vi "请求参数.vi"(10 "业务参数":T1, 11 "系统参数":T2) -> (3 "已排序的数组":T3[](array[typedef]))   [LabVIEW 2016, in "Alarm interface.lvlib" / "短信语音库.lvlib"]
uses:
  <vilib>/LVH/i3 OAuth/Controls/Name-Value Pair.ctl
  <vilib>/LVH/i3 OAuth/i3-oauth.lvlib
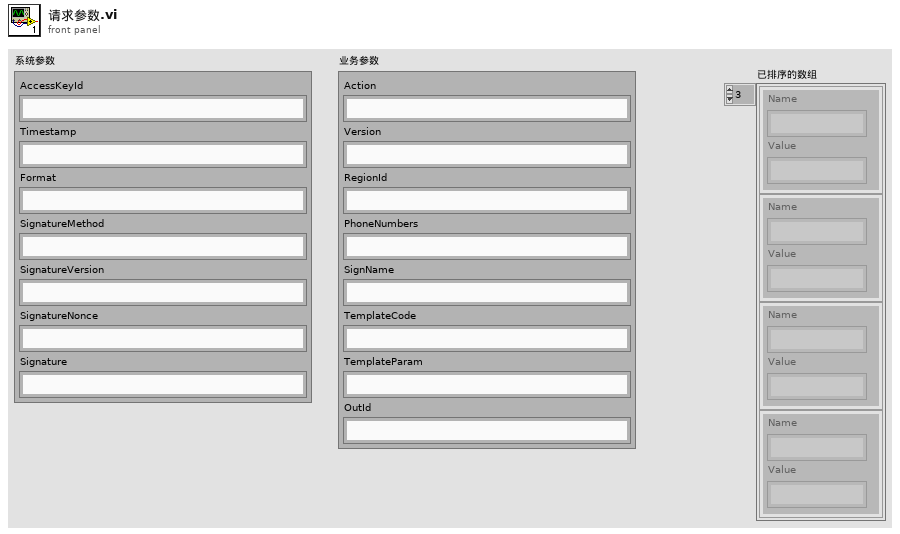
[diagram p1: front panel]
types:
  T1 = cluster{"Action":string, "Version":string, "RegionId":string, "PhoneNumbers":string, "SignName":string, "TemplateCode":string, "TemplateParam":string, "OutId":string}
  T2 = cluster{"AccessKeyId":string, "Timestamp":string, "Format":string, "SignatureMethod":string, "SignatureVersion":string, "SignatureNonce":string, "Signature":string}
  T3 = typedef "i3-oauth.lvlib/Name-Value Pair.ctl" = cluster{"Name":string, "Value":string}
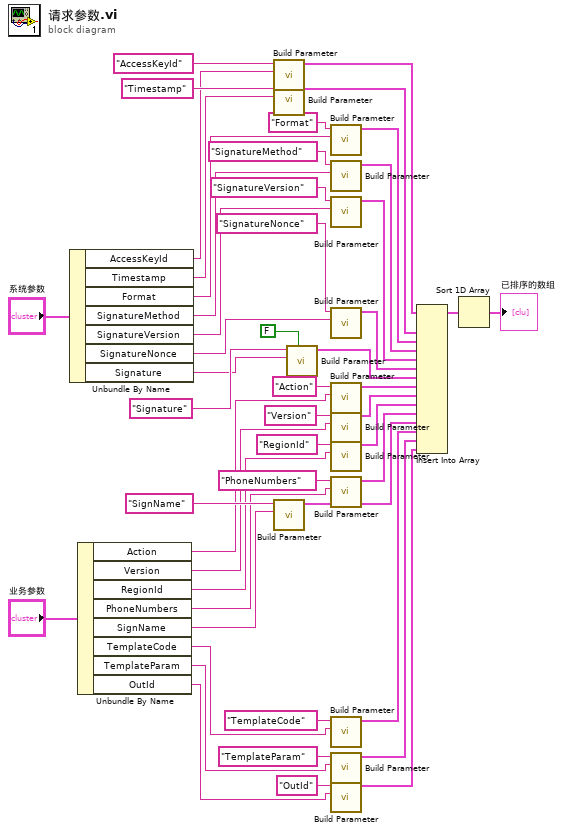
[diagram p0: block diagram]
diagram:
  n1 = Unbundle By Name("系统参数") -> ("AccessKeyId"=w25:string, "Timestamp"=w24:string, "Format"=w23:string, "SignatureMethod"=w22:string, "SignatureVersion"=w21:string, "SignatureNonce"=w20:string, "Signature"=w19:string)
  n2 = Unbundle By Name("业务参数") -> ("Action"=w14:string, "Version"=w13:string, "RegionId"=w12:string, "PhoneNumbers"=w11:string, "SignName"=w10:string, "TemplateCode"=w9:string, "TemplateParam"=w8:string, "OutId"=w7:string)
  n3 = call <vilib>:"Build Parameter.vi"("Value"=w25, "Key"="AccessKeyId") -> ("Parameter Array"=w35:T3[])  [unwired: 9 in]
  n4 = call <vilib>:"Build Parameter.vi"("Value"=w24, "Key"="Timestamp") -> ("Parameter Array"=w34:T3[])  [unwired: 9 in]
  n5 = call <vilib>:"Build Parameter.vi"("Value"=w10, "Key"="SignName") -> ("Parameter Array"=w4:T3[])  [unwired: 9 in]
  n6 = call <vilib>:"Build Parameter.vi"("Return Parameter? (T)"=FALSE, "Value"=w19, "Key"="Signature") -> ("Parameter Array"=w29:T3[])  [unwired: 8 in]
  n7 = call <vilib>:"Build Parameter.vi"("Value"=w23, "Key"="Format") -> ("Parameter Array"=w33:T3[])  [unwired: 9 in]
  n8 = call <vilib>:"Build Parameter.vi"("Value"=w22, "Key"="SignatureMethod") -> ("Parameter Array"=w32:T3[])  [unwired: 9 in]
  n9 = call <vilib>:"Build Parameter.vi"("Value"=w21, "Key"="SignatureVersion") -> ("Parameter Array"=w31:T3[])  [unwired: 9 in]
  n10 = call <vilib>:"Build Parameter.vi"("Value"=w20, "Key"="SignatureNonce") -> ("Parameter Array"=w30:T3[])  [unwired: 9 in]
  n11 = call <vilib>:"Build Parameter.vi"("Value"=w14, "Key"="Action") -> ("Parameter Array"=w18:T3[])  [unwired: 9 in]
  n12 = call <vilib>:"Build Parameter.vi"("Value"=w13, "Key"="Version") -> ("Parameter Array"=w17:T3[])  [unwired: 9 in]
  n13 = call <vilib>:"Build Parameter.vi"("Value"=w12, "Key"="RegionId") -> ("Parameter Array"=w16:T3[])  [unwired: 9 in]
  n14 = call <vilib>:"Build Parameter.vi"("Value"=w11, "Key"="PhoneNumbers") -> ("Parameter Array"=w5:T3[])  [unwired: 9 in]
  n15 = call <vilib>:"Build Parameter.vi"("Value"=w9, "Key"="TemplateCode") -> ("Parameter Array"=w3:T3[])  [unwired: 9 in]
  n16 = call <vilib>:"Build Parameter.vi"("Value"=w8, "Key"="TemplateParam") -> ("Parameter Array"=w2:T3[])  [unwired: 9 in]
  n17 = call <vilib>:"Build Parameter.vi"("Value"=w7, "Key"="OutId") -> ("Parameter Array"=w1:T3[])  [unwired: 9 in]
  n18 = Insert Into Array(array=w35, new element #1=w34, new element #2=w33, new element #3=w32, new element #4=w31, new element #5=w30, new element #6=w29, new element #7=w18, new element #8=w17, new element #9=w16, new element #10=w5, new element #11=w4, new element #12=w3, new element #13=w2, new element #14=w1) -> (w6:T3[])  [unwired: 1 in]
  n19 = Sort 1D Array(array=w6) -> (sorted array=→"已排序的数组":T3[])
